vi "frontPanel.vi"(8 "error in (no error)":errorcluster, 10 "ScriptEvent":refnum<class "ScriptEvent.lvclass">, 11 "ActionPanel in":refnum<class "rfAction.lvclass">) -> (0 "error out":errorcluster, 2 "ScriptEvent out":refnum<class "ScriptEvent.lvclass">, 3 "SingleToneAction out":refnum<class "rfAction.lvclass">)   [LabVIEW 2011, in "Views.lvlib" / "ScriptEditor.lvlib" / "rfAction.lvclass"]
uses:
  rfAction.lvclass
  Tools/Scripting/ScriptingEvent/ScriptEvent.lvclass
  rfAction.lvclass/rfAction.ctl
  Tools/Scripting/ScriptingEvent/ScriptEvents/Rf Event/rf.lvclass
  Tools/Scripting/ScriptingEvent/ScriptEvents/RfArray/rfArray.lvclass
  ActionPanel.lvclass
panel:
  in  "Current Phase (Degrees)":dbl format="%#.6g"
  in  "Phase (Degrees)":dbl format="%#.6g"
  out "editing":bool
  out "ready?":bool
  in  "close":bool
  in  "Frequency":dbl format="%#.6g"
  in  "States":u16(ring)
  in  "Amplitude":string
  in  "Dt":dbl format="%.6g"
  in  "Time":dbl format="%.6g"
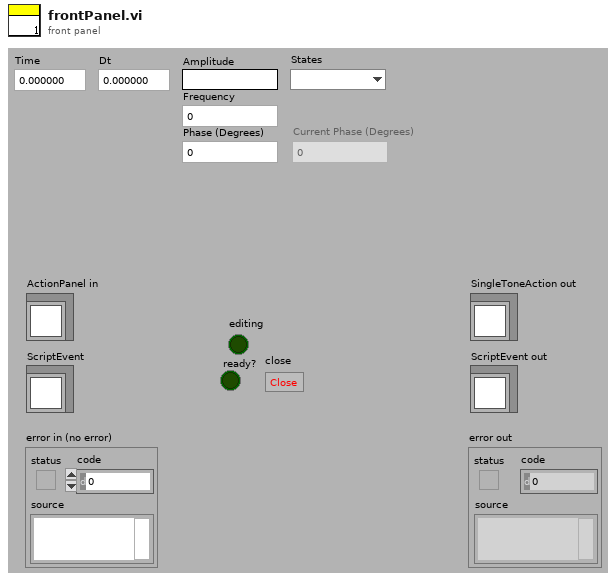
[diagram p1: front panel]
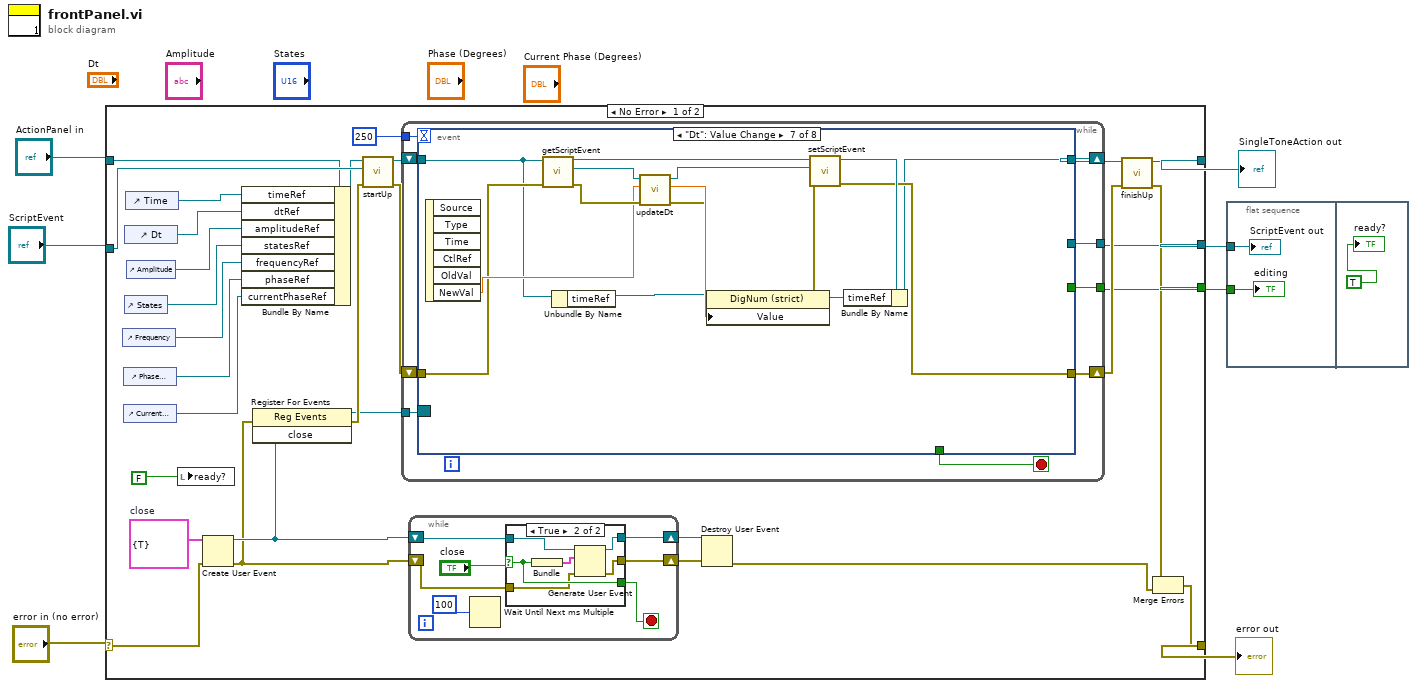
[diagram p0: block diagram]
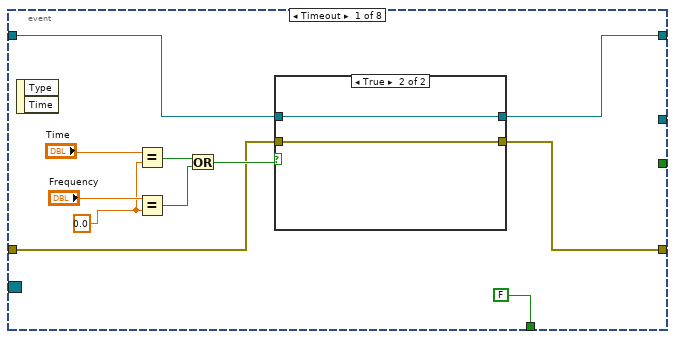
[diagram p3: hidden frame]
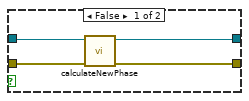
[diagram p4: hidden frame]
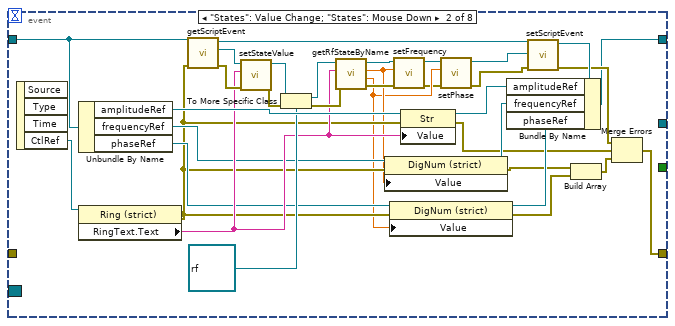
[diagram p5: hidden frame]
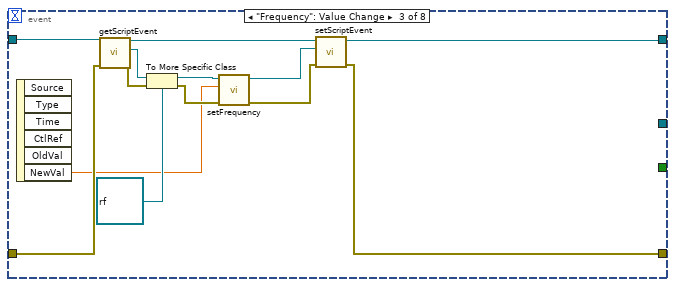
[diagram p6: hidden frame]
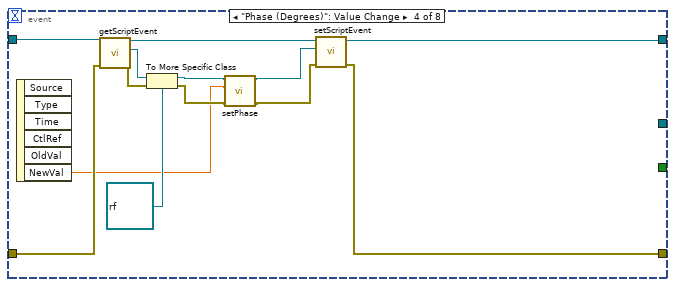
[diagram p7: hidden frame]
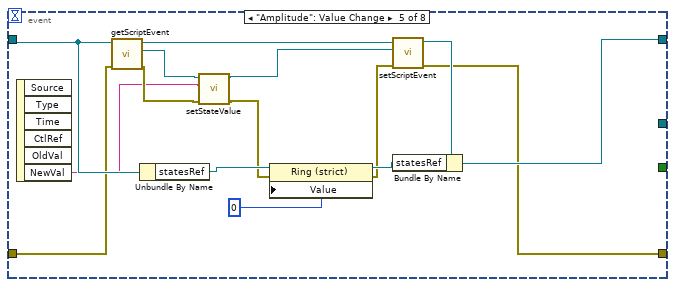
[diagram p8: hidden frame]
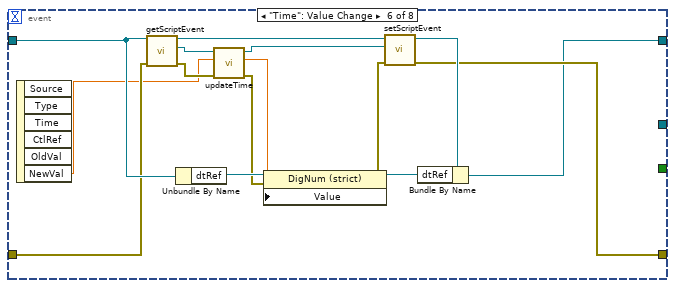
[diagram p9: hidden frame]
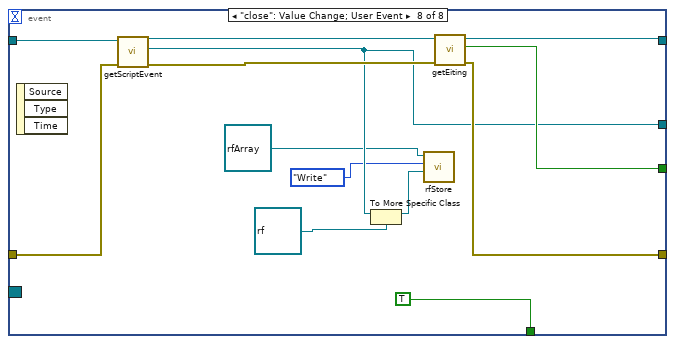
[diagram p10: hidden frame]
diagram:
  n1 = case shown="No Error" "error in (no error)" {
    selector: "error in (no error)" -> [w25 w198]
    tunnel: [w27 w198] -> w6
    tunnel: "ActionPanel in" -> [w17 w200]
    tunnel: [w37 w200] -> w4
    tunnel: "ScriptEvent" -> [w32 w199]
    tunnel: [w19 w199] -> w2
    tunnel: [w18 _] -> w1
    frame No Error {
      w26 = cluster{"close":bool} {"close"=TRUE}  # close
      n2 = control-ref of="Frequency"() -> (w10:refnum<vi>)
      n3 = control-ref of="Phase (Degrees)"() -> (w12:refnum<vi>)
      n4 = control-ref of="Current Phase (Degrees)"() -> (w9:refnum<vi>)
      n5 = control-ref of="Dt"() -> (w13:refnum<vi>)
      n6 = control-ref of="States"() -> (w11:refnum<vi>)
      n7 = control-ref of="Time"() -> (w15:refnum<vi>)
      n8 = control-ref of="Amplitude"() -> (w14:refnum<vi>)
      n9 = local write "ready?"(FALSE) -> ()
      n10 = Create User Event(user event datatype=w26, error in=w25) -> (user event=w24:refnum<user-event>, error out=w23:errorcluster)
      n11 = Bundle By Name(cluster=w17, "timeRef"=w15, "dtRef"=w13, "amplitudeRef"=w14, "statesRef"=w11, "frequencyRef"=w10, "phaseRef"=w12, "currentPhaseRef"=w9) -> (w16:refnum<class "rfAction.lvclass">)
      n12 = register-events(error in=w23, w24) -> (reference out=w21:refnum<event-registration>, error out=w22:errorcluster)  [unwired: 1 in]
      n13 = call-dynamic "startUp.vi"("error in (no error)"=w22, "ScriptEvent"=w32, "rfAction in"=w16) -> ("error out"=w34:errorcluster, "rfAction out"=w35:refnum<class "rfAction.lvclass">)  [unwired: 7 in]
      n14 = while {
        shift-right: [w62] -> w36
        shift-left: w35 -> [w61]
        shift-right: [w59] -> w33
        shift-left: w34 -> [w60]
        tunnel: w21 -> [w57]
        tunnel: [w56] -> w19
        tunnel: [w55] -> w18
        tunnel: 250 -> [w54]
        stop <- w58 stop-if-true
        n15 = event shown="[6] \"Dt\": Value Change" {
          selector: w57 -> [_ _ _ _ _ _ _ _]
          dyn-events: _ -> [_ _ _ _ _ _ _ _]
          timeout: w54 -> [_ _ _ _ _ _ _ _]
          tunnel: [w65 w105 w120 w133 w141 w157 w174 w194] -> w62
          tunnel: w61 -> [w66 w106 w126 w139 w144 w161 w171 w195]
          tunnel: w60 -> [w64 _ w123 w136 w142 w160 w172 w192]
          tunnel: [w63 w104 w121 w134 w140 w158 w175 w193] -> w59
          tunnel: [FALSE _ _ _ _ _ _ TRUE] -> w58
          tunnel: [_ _ _ _ _ _ _ w189] -> w56
          tunnel: [_ _ _ _ _ _ _ w191] -> w55
          event Timeout {
            w70 = 0.0
            n16 = event-data() -> ()  [unwired: 1 in, 2 out]
            n17 = Equal?(x="Time", y=w70) -> (x = y?=w69:bool)
            n18 = Equal?(x="Frequency", y=w70) -> (x = y?=w68:bool)
            n19 = Or(x=w69, y=w68) -> (x .or. y?=w67:bool)
            n20 = case shown="True" w67 {
              tunnel: w66 -> [w77 w79]
              tunnel: [w76 w79] -> w65
              tunnel: w64 -> [w75 w78]
              tunnel: [w74 w78] -> w63
              frame False {
                n21 = call "calculateNewPhase.vi"("error in (no error)"=w75, "rfAction in"=w77) -> ("error out"=w74:errorcluster, "rfAction out"=w76:refnum<class "rfAction.lvclass">)  [unwired: 8 in]
              }
              frame True {
              }
            }
          }
          event "States": Value Change; "States": Mouse Down {
            n22 = event-data() -> ("CtlRef"=w103:refnum<vi>)  [unwired: 1 in, 3 out]
            n23 = Unbundle By Name(w106) -> ("amplitudeRef"=w110:refnum<vi>, "frequencyRef"=w96:refnum<vi>, "phaseRef"=w95:refnum<vi>)
            n24 = property class="Ring (strict)"(reference=w103) -> (error out=w94:errorcluster, "RingText.Text"=w97:string)  [unwired: 1 in, 1 out]
            n25 = call "getScriptEvent.vi"("error in (no error)"=w94, "ActionPanel.lvclass in"=w106) -> ("error out"=w111:errorcluster, "ScriptEvent.lvclass"=w112:refnum<class "ScriptEvent.lvclass">, "ActionPanel.lvclass out"=w113:refnum<class "rfAction.lvclass">)  [unwired: 7 in]
            n26 = call "setStateValue.vi"("error in (no error)"=w111, "stateValue"=w97, "ScriptEvent in"=w112) -> ("error out"=w101:errorcluster, "ScriptEvent out"=w102:refnum<class "ScriptEvent.lvclass">)  [unwired: 7 in]
            n27 = To More Specific Class(target class=refnum<class "rf.lvclass"> refnum ("Tools.lvlib:Scripting.lvlib:rf.lvclass"), reference=w102, error in=w101) -> (specific class reference=w100:refnum<class "rf.lvclass">, error out=w98:errorcluster)
            n28 = call "getRfStateByName.vi"("error in (no error)"=w98, "stateName"=w97, "rf in"=w100) -> ("error out"=w86:errorcluster, "phase"=w83:dbl, "frequency"=w85:dbl, "rf out"=w87:refnum<class "rf.lvclass">)  [unwired: 5 in]
            n29 = property class="DigNum (strict)"(reference=w96, error in=w94, "Value"=w85) -> (reference out=w93:refnum<vi>, error out=w91:errorcluster)
            n30 = property class="DigNum (strict)"(reference=w95, error in=w94, "Value"=w83) -> (reference out=w92:refnum<vi>, error out=w90:errorcluster)
            n31 = call "setFrequency.vi"("error in (no error)"=w86, "frequency"=w85, "rf in"=w87) -> ("error out"=w82:errorcluster, "rf out"=w84:refnum<class "rf.lvclass">)  [unwired: 7 in]
            n32 = property class="Str"(reference=w110, error in=w94, "Value"=w97) -> (reference out=w109:refnum<vi>, error out=w89:errorcluster)
            n33 = call "setPhase.vi"("error in (no error)"=w82, "phase"=w83, "rf in"=w84) -> ("error out"=w80:errorcluster, "rf out"=w81:refnum<class "rf.lvclass">)  [unwired: 7 in]
            n34 = call "setScriptEvent.vi"("error in (no error)"=w80, "ScriptEvent.lvclass"=w81, "ActionPanel.lvclass in"=w113) -> ("error out"=w107:errorcluster, "ActionPanel.lvclass out"=w108:refnum<class "rfAction.lvclass">)  [unwired: 7 in]
            n35 = Bundle By Name(cluster=w108, "amplitudeRef"=w109, "frequencyRef"=w93, "phaseRef"=w92) -> (w105:refnum<class "rfAction.lvclass">)
            n36 = Build Array(w91, w90) -> (w88:errorcluster[])
            n37 = Merge Errors(w107, w89, w88) -> (w104:errorcluster)
          }
          event "Frequency": Value Change {
            n38 = event-data() -> ("NewVal"=w114:dbl)  [unwired: 1 in, 5 out]
            n39 = call "getScriptEvent.vi"("error in (no error)"=w123, "ActionPanel.lvclass in"=w126) -> ("error out"=w124:errorcluster, "ScriptEvent.lvclass"=w125:refnum<class "ScriptEvent.lvclass">, "ActionPanel.lvclass out"=w122:refnum<class "rfAction.lvclass">)  [unwired: 7 in]
            n40 = To More Specific Class(target class=refnum<class "rf.lvclass"> refnum ("Tools.lvlib:Scripting.lvlib:rf.lvclass"), reference=w125, error in=w124) -> (specific class reference=w116:refnum<class "rf.lvclass">, error out=w115:errorcluster)
            n41 = call "setFrequency.vi"("error in (no error)"=w115, "frequency"=w114, "rf in"=w116) -> ("error out"=w118:errorcluster, "rf out"=w117:refnum<class "rf.lvclass">)  [unwired: 7 in]
            n42 = call "setScriptEvent.vi"("error in (no error)"=w118, "ScriptEvent.lvclass"=w117, "ActionPanel.lvclass in"=w122) -> ("error out"=w121:errorcluster, "ActionPanel.lvclass out"=w120:refnum<class "rfAction.lvclass">)  [unwired: 7 in]
          }
          event "Phase (Degrees)": Value Change {
            n43 = event-data() -> ("NewVal"=w127:dbl)  [unwired: 1 in, 5 out]
            n44 = call "getScriptEvent.vi"("error in (no error)"=w136, "ActionPanel.lvclass in"=w139) -> ("error out"=w137:errorcluster, "ScriptEvent.lvclass"=w138:refnum<class "ScriptEvent.lvclass">, "ActionPanel.lvclass out"=w135:refnum<class "rfAction.lvclass">)  [unwired: 7 in]
            n45 = To More Specific Class(target class=refnum<class "rf.lvclass"> refnum ("Tools.lvlib:Scripting.lvlib:rf.lvclass"), reference=w138, error in=w137) -> (specific class reference=w132:refnum<class "rf.lvclass">, error out=w130:errorcluster)
            n46 = call "setPhase.vi"("error in (no error)"=w130, "phase"=w127, "rf in"=w132) -> ("error out"=w129:errorcluster, "rf out"=w131:refnum<class "rf.lvclass">)  [unwired: 7 in]
            n47 = call "setScriptEvent.vi"("error in (no error)"=w129, "ScriptEvent.lvclass"=w131, "ActionPanel.lvclass in"=w135) -> ("error out"=w134:errorcluster, "ActionPanel.lvclass out"=w133:refnum<class "rfAction.lvclass">)  [unwired: 7 in]
          }
          event "Amplitude": Value Change {
            n48 = event-data() -> ("NewVal"=w143:string)  [unwired: 1 in, 5 out]
            n49 = call "getScriptEvent.vi"("error in (no error)"=w142, "ActionPanel.lvclass in"=w144) -> ("error out"=w146:errorcluster, "ScriptEvent.lvclass"=w148:refnum<class "ScriptEvent.lvclass">, "ActionPanel.lvclass out"=w154:refnum<class "rfAction.lvclass">)  [unwired: 7 in]
            n50 = Unbundle By Name(w144) -> ("statesRef"=w153:refnum<vi>)
            n51 = call "setStateValue.vi"("error in (no error)"=w146, "stateValue"=w143, "ScriptEvent in"=w148) -> ("error out"=w145:errorcluster, "ScriptEvent out"=w147:refnum<class "ScriptEvent.lvclass">)  [unwired: 7 in]
            n52 = property class="Ring (strict)"(reference=w153, error in=w145, "Value"=0) -> (reference out=w150:refnum<vi>, error out=w149:errorcluster)
            n53 = call "setScriptEvent.vi"("error in (no error)"=w149, "ScriptEvent.lvclass"=w147, "ActionPanel.lvclass in"=w154) -> ("error out"=w140:errorcluster, "ActionPanel.lvclass out"=w151:refnum<class "rfAction.lvclass">)  [unwired: 7 in]
            n54 = Bundle By Name(cluster=w151, "statesRef"=w150) -> (w141:refnum<class "rfAction.lvclass">)
          }
          event "Time": Value Change {
            n55 = event-data() -> ("NewVal"=w159:dbl)  [unwired: 1 in, 5 out]
            n56 = call "getScriptEvent.vi"("error in (no error)"=w160, "ActionPanel.lvclass in"=w161) -> ("error out"=w167:errorcluster, "ScriptEvent.lvclass"=w168:refnum<class "ScriptEvent.lvclass">, "ActionPanel.lvclass out"=w169:refnum<class "rfAction.lvclass">)  [unwired: 7 in]
            n57 = Unbundle By Name(w161) -> ("dtRef"=w166:refnum<vi>)
            n58 = call "updateTime.vi"("error in (no error)"=w167, "time"=w159, "ScriptEvent in"=w168) -> ("error out"=w155:errorcluster, "dt"=w165:dbl, "ScriptEvent out"=w156:refnum<class "ScriptEvent.lvclass">)  [unwired: 6 in]
            n59 = property class="DigNum (strict)"(reference=w166, error in=w155, "Value"=w165) -> (reference out=w164:refnum<vi>, error out=w162:errorcluster)
            n60 = call "setScriptEvent.vi"("error in (no error)"=w162, "ScriptEvent.lvclass"=w156, "ActionPanel.lvclass in"=w169) -> ("error out"=w158:errorcluster, "ActionPanel.lvclass out"=w163:refnum<class "rfAction.lvclass">)  [unwired: 7 in]
            n61 = Bundle By Name(cluster=w163, "dtRef"=w164) -> (w157:refnum<class "rfAction.lvclass">)
          }
          event "Dt": Value Change {
            n62 = event-data() -> ("NewVal"=w173:dbl)  [unwired: 1 in, 5 out]
            n63 = call "getScriptEvent.vi"("error in (no error)"=w172, "ActionPanel.lvclass in"=w171) -> ("error out"=w179:errorcluster, "ScriptEvent.lvclass"=w180:refnum<class "ScriptEvent.lvclass">, "ActionPanel.lvclass out"=w184:refnum<class "rfAction.lvclass">)  [unwired: 7 in]
            n64 = Unbundle By Name(w171) -> ("timeRef"=w170:refnum<vi>)
            n65 = call "updateDt.vi"("error in (no error)"=w179, "dt"=w173, "ScriptEvent in"=w180) -> ("error out"=w177:errorcluster, "time"=w178:dbl, "ScriptEvent out"=w176:refnum<class "ScriptEvent.lvclass">)  [unwired: 6 in]
            n66 = property class="DigNum (strict)"(reference=w170, error in=w177, "Value"=w178) -> (reference out=w183:refnum<vi>, error out=w181:errorcluster)
            n67 = call "setScriptEvent.vi"("error in (no error)"=w181, "ScriptEvent.lvclass"=w176, "ActionPanel.lvclass in"=w184) -> ("error out"=w175:errorcluster, "ActionPanel.lvclass out"=w182:refnum<class "rfAction.lvclass">)  [unwired: 7 in]
            n68 = Bundle By Name(cluster=w182, "timeRef"=w183) -> (w174:refnum<class "rfAction.lvclass">)
          }
          event "close": Value Change; User Event {
            n69 = event-data() -> ()  [unwired: 1 in, 3 out]
            n70 = call "getScriptEvent.vi"("error in (no error)"=w192, "ActionPanel.lvclass in"=w195) -> ("error out"=w196:errorcluster, "ScriptEvent.lvclass"=w189:refnum<class "ScriptEvent.lvclass">, "ActionPanel.lvclass out"=w197:refnum<class "rfAction.lvclass">)  [unwired: 7 in]
            n71 = To More Specific Class(target class=refnum<class "rf.lvclass"> refnum ("Tools.lvlib:Scripting.lvlib:rf.lvclass"), reference=w189) -> (specific class reference=w185:refnum<class "rf.lvclass">)  [unwired: 1 in, 1 out]
            n72 = call "rfStore.vi"("rf.lvclass"=w185, "action"=enum16{"Write", "Read"}."Write", "rfArray in"=refnum<class "rfArray.lvclass"> refnum ("Tools.lvlib:Scripting.lvlib:rfArray.lvclass")) -> ()  [unwired: 5 in, 4 out]
            n73 = call "getEiting.vi"("error in (no error)"=w196, "ActionPanel.lvclass in"=w197) -> ("error out"=w193:errorcluster, "editing?"=w191:bool, "ActionPanel.lvclass out"=w194:refnum<class "rfAction.lvclass">)  [unwired: 7 in]
          }
        }
      }
      n74 = while {
        shift-right: [w41] -> w30
        shift-left: w23 -> [w40]
        shift-right: [w42] -> w31
        shift-left: w24 -> [w44]
        stop <- w43 stop-if-true
        n75 = Wait Until Next ms Multiple(millisecond multiple=100) -> ()  [unwired: 1 out]
        n76 = case shown="True" "close" {
          selector: "close" -> [w47 w51]
          tunnel: w44 -> [w46 w53]
          tunnel: [w47 w51] -> w43
          tunnel: [w46 w50] -> w42
          tunnel: [w45 w49] -> w41
          tunnel: w40 -> [w45 w48]
          frame False {
          }
          frame True {
            n77 = Bundle(w51) -> (w52:cluster{bool})  [unwired: 1 in]
            n78 = Generate User Event(user event=w53, event data cluster=w52, error in=w48) -> (user event out=w50:refnum<user-event>, error out=w49:errorcluster)
          }
        }
      }
      n79 = Destroy User Event(user event=w31, error in=w30) -> (error out=w28:errorcluster)
      n80 = call-dynamic "finishUp.vi"("error in (no error)"=w33, "rfAction in"=w36) -> ("error out"=w29:errorcluster, "rfAction out"=w37:refnum<class "rfAction.lvclass">)  [unwired: 8 in]
      n81 = Merge Errors(w29, w28) -> (w27:errorcluster)
    }
    frame Error {
    }
  }
  "error out" <- w6
  "SingleToneAction out" <- w4
  n82 = flat-sequence {
    tunnel: w2 -> [w202]
    tunnel: w1 -> [w201]
    frame #0 {
      "ScriptEvent out" <- w202
      "editing" <- w201
    }
    frame #1 {
      "ready?" <- TRUE
    }
  }
